vi "Get Lifecycle State for Process.vi"(10 "Process":string, 11 "Debug State Analyzer In":refnum<class "Debug State Analyzer.lvclass">) -> (2 "Lifecycle State":string, 3 "Debug State Analyzer Out":refnum<class "Debug State Analyzer.lvclass">)   [LabVIEW 2020, in "Debug State Analyzer.lvclass"]
uses:
  Debug State Analyzer.lvclass
  Debug State Analyzer.lvclass/Debug State Analyzer.ctl
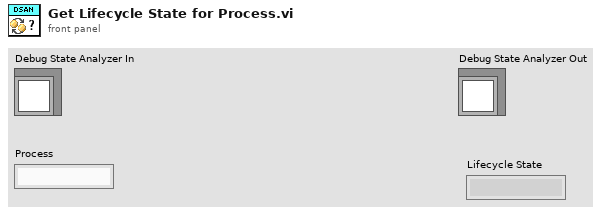
[diagram p1: front panel]
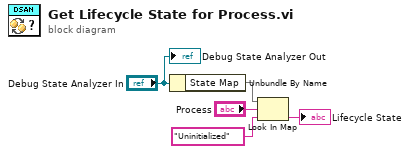
[diagram p0: block diagram]
diagram:
  n1 = Unbundle By Name("Debug State Analyzer In") -> ("State Map"=w4:map{string, string})
  n2 = Look In Map(map=w4, key="Process", default value="Uninitialized") -> (value=→"Lifecycle State":string)  [unwired: 1 out]
  "Debug State Analyzer Out" <- "Debug State Analyzer In"
